vi "LuaVIEW Check Synopsis_srv.vi"(7 "certificate":string, 11 "synopsis":string) -> (4 "synopsis error":string, 15 "error out":errorcluster)   [LabVIEW 2012]
uses:
  clientsrv/typedefs/t_ClientSrv Access Levels.ctl
  typedefs/et_LuaVIEW CIN Actions.ctl
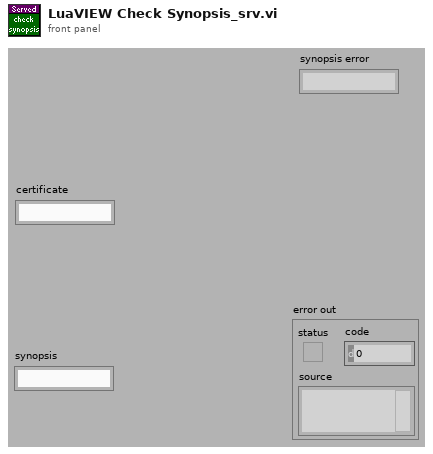
[diagram p1: front panel]
types:
  T1 = typedef "t_ClientSrv Access Levels.ctl" = enum16{"observer", "operator", "local"}
  T2 = typedef "et_LuaVIEW CIN Actions.ctl" = enum16{"checksynopsis", "_open", "_registerpublic", "_registerexport", "__never_an_error_result_ns", "luaversion", "cinversion", "_totals", "_taskcount", "pathological", "_unregnextpublic", "registryusecount", "__per_state_actions", "regsetprivate", "regsetindex", "regsetmodule", "_revokeexports", "_usepublic", "prepare", "compile", "execute", "call", "unregstaterefs", "_close", "pullboolean", "pullnumber", "pullI8", "pullU8", "pullI16", "pullU16", "pullI32", "pullU32", "pullobject", "pullrefnum", "pullstring", "pullflat", "pushflat", "pushobject", "getattribute", "setattribute", "stacktostring", "_startyieldtest", "_endyieldtest", "_pollprintbuffer", "__never_an_error_result_ps", "_pollexport", "setclone", "forcecleanup", "gettop", "clearstack", "insert", "pushboolean", "pushnumber", "pushrefnum", "pushstring", "pushnil", "pushvalue", "gettaskref", "settaskref"}
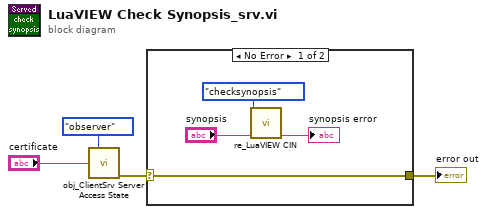
[diagram p0: block diagram]
diagram:
  n1 = call "obj_ClientSrv Server Access State.vi"("access level"=t_ClientSrv_Access_Levels."observer", "certificate in"="certificate") -> ("error out"=w1:errorcluster)  [unwired: 11 in, 2 out]
  n2 = case shown="No Error" w1 {
    selector: w1 -> [w8 w9]
    tunnel: [w8 w9] -> w2
    frame No Error {
      n3 = call "re_LuaVIEW CIN.vi"("action"=et_LuaVIEW_CIN_Actions."checksynopsis", "string in"="synopsis") -> ("string out"=→"synopsis error":string)  [unwired: 7 in, 6 out]
    }
    frame Error {
    }
  }
  "error out" <- w2
